vi "Host to Target - Host.vi"() -> ()   [LabVIEW 2010]
uses:
  <vilib>/userDefined/High Color/nirio_resource_hc.ctl
  <vilib>/rvi/interface/nirviOpenFPGA/nirviOpenFPGA.xnode
  Host to Target - FPGA.vi
  <vilib>/rvi/interface/nirviOpenFPGA/nirviOpenFPGA.ctl
  <vilib>/rvi/interface/nirviOpenFPGA/nirviopenstate.ctl
  <vilib>/picture/picture.llb/imagedata.ctl
  <vilib>/rvi/interface/common/nirviIntfCommonState.ctl
  <vilib>/rvi/interface/common/nirviIntfModes.ctl
  Program Files/National Instruments/LabVIEW 2010/resource/RVI/emulation/niLvFpgaEmulationMode.ctl
  <vilib>/eio/XNode/Errors/EIOXNodeErrorStruct.ctl
  <vilib>/eio/XNode/Errors/EIOXNodeInternalErrorTypes.ctl
  <vilib>/eio/XNode/Errors/EIOXNodeUserErrorTypes.ctl
  <vilib>/XNodeSupport/XNodeRect32.ctl
  <vilib>/XNodeSupport/XNodeInt.ctl
  <vilib>/XNodeSupport/XNodeTerms.ctl
  <vilib>/XNodeSupport/XNodeTerm.ctl
  <vilib>/XNodeSupport/XNodeString.ctl
  <vilib>/XNodeSupport/XNodeVariant.ctl
  <vilib>/XNodeSupport/XNodeBool.ctl
  <vilib>/rvi/interface/nirviMethod/nirviMethod.xnode
  <vilib>/rvi/interface/common/niFpgaNodeNameForErrorReporting.ctl
  <vilib>/rvi/interface/nirviReadWriteControl/nirviReadWriteControl.xnode
  <vilib>/rvi/interface/nirviCloseFPGA/nirviCloseFPGA.xnode
  <vilib>/rvi/interface/RandomDataEmulation/nirviRandomDataOpen.vi
  <vilib>/rvi/interface/RandomDataEmulation/nirviRandomDataRunMethod.vi
  <vilib>/rvi/interface/RandomDataEmulation/nirviRandomDataDMAMethods.vi
  <vilib>/rvi/interface/RandomDataEmulation/nirviRandomDataWaitOnIRQMethod.vi
  <vilib>/rvi/interface/RandomDataEmulation/nirviRandomDataAcknowledgeIRQMethod.vi
  <vilib>/rvi/interface/RandomDataEmulation/nirviRandomDataClose.vi
  <vilib>/XNodeSupport/NI_XNodeSupport.lvlib
panel:
  in  "Write Period (msec)":u32=500
  out "Reading":bool
  out "Writing":bool
  out "Host to Target FIFO":u32(slide) step=416361304 scale=0.0..21.0
  in  "Stop":bool
  in  "Read Period(mSec)":u32=250
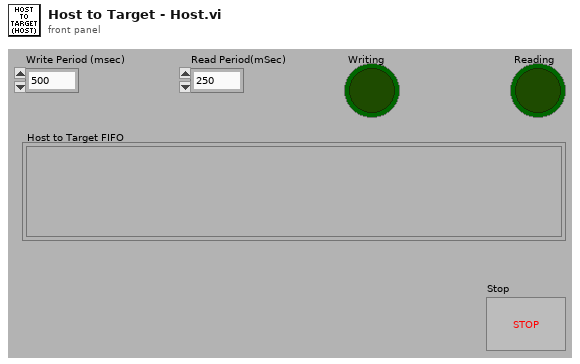
[diagram p1: front panel]
types:
  T1 = typedef "niFpgaNodeNameForErrorReporting.ctl" = enum16{"Open FPGA VI Reference", "Read/Write Control", "Invoke Method: Abort", "Invoke Method: Acknowledge IRQ", "Invoke Method: Download", "Invoke Method: FIFO.Configure", "Invoke Method: FIFO.Read", "Invoke Method: FIFO.Start", "Invoke Method: FIFO.Stop", "Invoke Method: FIFO.Write", "Invoke Method: Reset", "Invoke Method: Run", "Invoke Method: Wait on IRQ", "Close FPGA VI Reference"}
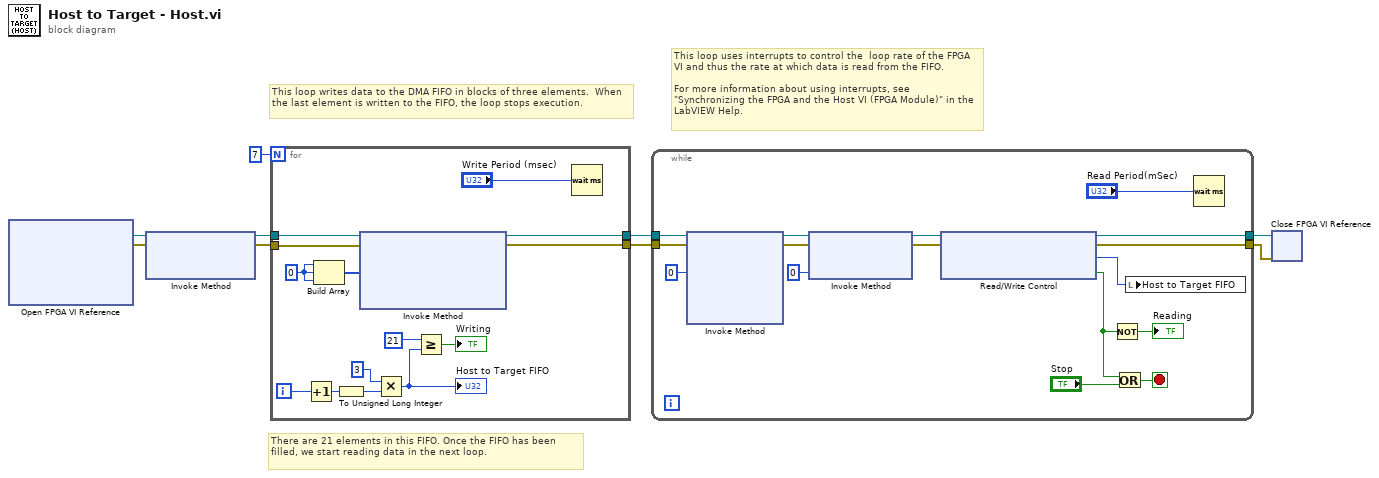
[diagram p0: block diagram]
diagram:
  # "There are 21 elements in this FIFO. Once the FIFO has been filled, we start reading data in the next loop."
  # "This loop writes data to the DMA FIFO in blocks of three elements.  When the last element is written to the FIFO, the loop stops execution."
  # "This loop uses interrupts to control the  loop rate of the FPGA VI and thus the rate at which data is read from the FIFO.\n\nFor more information about using interrupts, see \"Synchronizing the FPGA and the Host VI (FPGA Module)\" in the LabVIEW Help."
  n1 = xnode "Open FPGA VI Reference"() -> ("FPGA VI Reference Out"=w2:refnum<k20>, "error out"=w1:errorcluster)  [unwired: 2 in]
  n2 = xnode "Invoke Method"("FPGA VI Reference In"=w2, "error in"=w1) -> ("FPGA VI Reference Out"=w4:refnum<k20>, "error out"=w3:errorcluster)  [unwired: 1 in]
  n3 = for {
    N: 7 -> [_]
    tunnel: w4 -> [w22]
    tunnel: w3 -> [w21]
    tunnel: [w18] -> w6
    tunnel: [w17] -> w5
    i -> [w16]
    w20 = i16 0 ("Data")
    n4 = Increment(x=w16) -> (x+1=w13:i32)
    n5 = Build Array(w20, w20, w20) -> (w19:i16[])
    n6 = To Unsigned Long Integer(number=w13) -> (unsigned 32bit integer=w15:u32)
    n7 = xnode "Invoke Method"("FPGA VI Reference In"=w22, "error in"=w21, "Data"=w19) -> ("FPGA VI Reference Out"=w18:refnum<k20>, "error out"=w17:errorcluster)  [unwired: 1 in, 1 out]
    n8 = Multiply(x=u32 3, y=w15) -> (x*y=w10:u32)
    "Host to Target FIFO" <- w10
    n9 = Greater Or Equal?(x=u32 21 ("y"), y=w10) -> (x >= y?=→"Writing":bool)
    n10 = Wait (ms)(milliseconds to wait="Write Period (msec)") -> ()  [unwired: 1 out]
  }
  n11 = while {
    tunnel: w6 -> [w47]
    tunnel: w5 -> [w45]
    tunnel: [w49] -> w8
    tunnel: [w48] -> w7
    stop <- w50 stop-if-true
    n12 = xnode "Invoke Method"("FPGA VI Reference In"=w47, "error in"=w45, "IRQ Number(s)"=0) -> ("FPGA VI Reference Out"=w44:refnum<k20>, "error out"=w43:errorcluster)  [unwired: 1 in, 2 out]
    n13 = xnode "Invoke Method"("FPGA VI Reference In"=w44, "error in"=w43, "IRQ Number(s)"=0) -> ("FPGA VI Reference Out"=w42:refnum<k20>, "error out"=w41:errorcluster)
    n14 = xnode "Read/Write Control"("FPGA VI Reference In"=w42, "error in"=w41) -> ("FPGA VI Reference Out"=w49:refnum<k20>, "error out"=w48:errorcluster, "Number of Elements to Read"=w35:u32, "Timed Out?"=w36:bool)
    n15 = Not(x=w36) -> (.not. x?=→"Reading":bool)
    n16 = Or(x=w36, y="Stop") -> (x .or. y?=w50:bool)
    n17 = local write "Host to Target FIFO"(w35) -> ()
    n18 = Wait (ms)(milliseconds to wait="Read Period(mSec)") -> ()  [unwired: 1 out]
  }
  n19 = xnode "Close FPGA VI Reference"("FPGA VI Reference In"=w8, "error in"=w7) -> ()  [unwired: 1 out]
